vi "SetWindowSurfaceVSync.vi"(8 "No Error":errorcluster, 10 "VSync":T1 items=["SDL_WINDOW_SURFACE_VSYNC_DISABLED"=0, "SDL_WINDOW_SURFACE_VSYNC_ADAPTIVE"=-1], 11 "Window [SDL_Window *]":T2 format="%.0x") -> (0 "Error Out":errorcluster)   [LabVIEW 2026, in "SDL3.lvlib" / "Video.lvlib"]
doc: "<B>Summary</B>\nToggle VSync for the window surface.\n\n<B>Remarks</B>\nWhen a window surface is created, vsync defaults to <B>SDL_WINDOW_SURFACE_VSYNC_DISABLED</B>.\n\nThe vsync parameter can be 1 to synchronize present with every vertical refresh, 2 to synchronize present with every second vertical refresh, etc., <B>SDL_WINDOW_SURFACE_VSYNC_ADAPTIVE</B> for late swap tearing (adaptive vsync), or <B>SDL_WINDOW_SURFACE_VSYNC_DISABLED</B> to disable. Not every value is supported by every driver, so you should check the return value to see whether the requested setting is supported."
uses:
  Video.lvlib
  VSync--ring.ctl
  <vilib>/Utility/error.llb/Error Cluster From Error Code.vi
  Error/Error.lvlib
  Lib/SDL3.dll
  SDL_Window--pointer.ctl
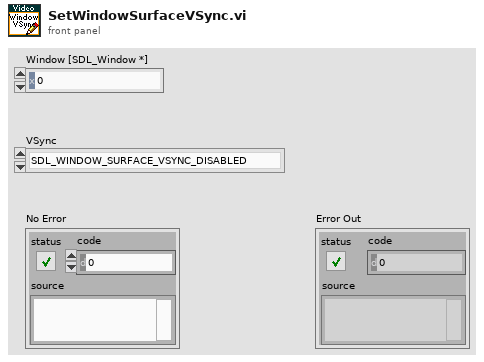
[diagram p1: front panel]
types:
  T1 = typedef "SDL3.lvlib/Video.lvlib/VSync--ring.ctl" = i32
  T2 = typedef "SDL3.lvlib/Video.lvlib/SDL_Window--pointer.ctl" = i64
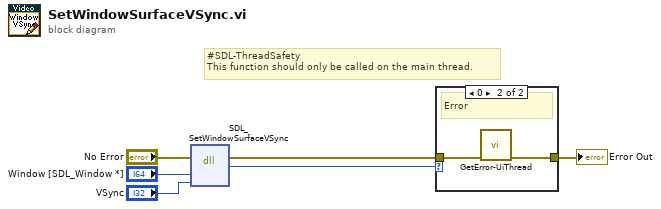
[diagram p0: block diagram]
diagram:
  # "#SDL-ThreadSafety\nThis function should only be called on the main thread."
  n1 = dll-call lib="C:/Users/saukko/Dev/LV-SDL3/Sources/SDL3/Lib/SDL3.*" fn="SDL_SetWindowSurfaceVSync"(error in="No Error", "window"="Window [SDL_Window *]", "vsync"="VSync") -> (error out=w3:errorcluster, "return type"=w2:i32)  [unwired: 4 in, 1 out]
  n2 = case shown="0" w2 {
    tunnel: w3 -> [w7 w9]
    tunnel: [w7 w8] -> w5
    frame Default {
      # "Ok"
    }
    frame 0 {
      # "Error"
      n3 = call "GetError-UiThread.vi"("No Error"=w9) -> ("error out"=w8:errorcluster)  [unwired: 10 in]
    }
  }
  "Error Out" <- w5
